vi "Filter-Compute Scale Factor.vi"(0 "Filter":T1 {"IIR Filter Cluster"."Forward Coefficients" format="%.4f"; "IIR Filter Cluster"."Reverse Coefficients" format="%.4f"}, 7 "Sampling Rate (Hz)":dbl, 11 "error in (no error)":errorcluster) -> (4 "Filter out":T1 {"IIR Filter Cluster"."Forward Coefficients" format="%.4f"; "IIR Filter Cluster"."Reverse Coefficients" format="%.4f"}, 15 "error out":errorcluster)   [LabVIEW 2020]
uses:
  Controls/Filter XCtl/Filter Data.ctl
  Controls/Filter XCtl/Filter XCtl.xctl
panel:
  out "RMS":dbl
  out "Scale Factor":dbl
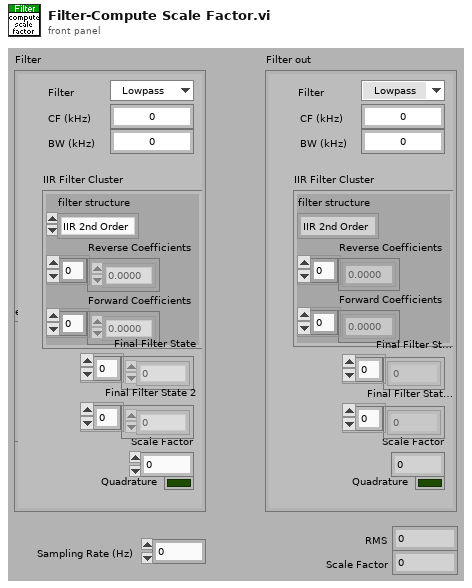
[diagram p1: front panel]
types:
  T1 = typedef "Filter XCtl.xctl/Filter Data.ctl" = cluster{"CF (kHz)":dbl, "BW (kHz)":dbl, "IIR Filter Cluster":cluster{"filter structure":enum32{"IIR 2nd Order", "IIR 4th Order"}, "Reverse Coefficients":dbl[], "Forward Coefficients":dbl[]}, "Final Filter State":dbl[], "Scale Factor":dbl, "Final Filter State 2":dbl[], "Quadrature":bool, "Type":enum16{"Lowpass", "Highpass", "Bandpass", "Bandstop", "OFF"}}
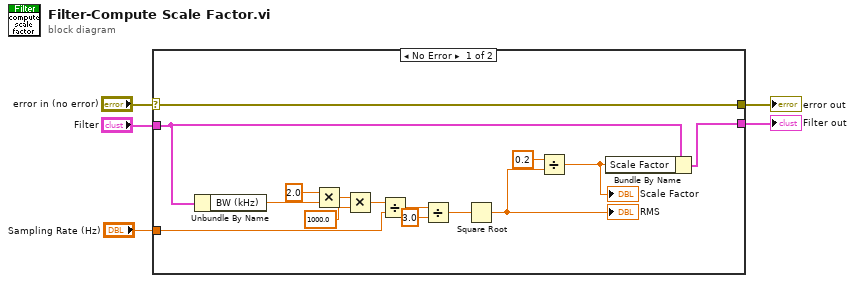
[diagram p0: block diagram]
diagram:
  n1 = case shown="No Error" "error in (no error)" {
    selector: "error in (no error)" -> [w18 w22]
    tunnel: "Filter" -> [w20 w21]
    tunnel: [w19 w21] -> w4
    tunnel: [w18 w22] -> w2
    tunnel: "Sampling Rate (Hz)" -> [w10 _]
    frame No Error {
      n2 = Unbundle By Name(w20) -> ("BW (kHz)"=w15:dbl)
      n3 = Multiply(x=2.0, y=w15) -> (x*y=w13:dbl)
      n4 = Multiply(x=w13, y=1000.0) -> (x*y=w11:dbl)
      n5 = Divide(x=w11, y=w10) -> (x/y=w9:dbl)
      n6 = Divide(x=w9, y=3.0) -> (x/y=w7:dbl)
      n7 = Square Root(x=w7) -> (sqrt(x)=w6:dbl)
      "RMS" <- w6
      n8 = Divide(x=0.2, y=w6) -> (x/y=w16:dbl)
      "Scale Factor" <- w16
      n9 = Bundle By Name(cluster=w20, "Scale Factor"=w16) -> (w19:T1)
    }
    frame Error {
    }
  }
  "error out" <- w2
  "Filter out" <- w4
